vi "getConfiguration.vi"(8 "error in (no error)":errorcluster, 11 "Xcite in":refnum<class "Xcite.lvclass">) -> (0 "error out":errorcluster, 2 "configuration":cluster{"intensities":u32[], "on_states":u8[]}, 3 "Xcite out":refnum<class "Xcite.lvclass">)   [LabVIEW 2019, in "Xcite.lvclass"]
doc: "Returns the on/off state and intensity of each channel."
uses:
  Xcite.lvclass
  Xcite.lvclass/Xcite.ctl
  etc.xcite/XCite.lvlib
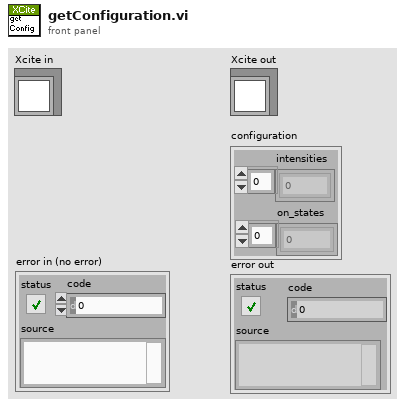
[diagram p1: front panel]
types:
  T1 = cluster{"LightSourceName":string, "hDevice":u64, "hCamera":u64, "iNumChannels":i32, "iNumWheels":i32, "dwSystemState":u32, "dwSerialNumber":u32, "dwSystemCaps":u32, "iLastChannelOnWheel":i16[], "XCiteChannels":cluster{"szLedName":string, "iWaveLength":i32, "IBelongToWheelNumber":i32, "iIntensity":i32, "iIntensityMin":i32, "iIntensityMax":i32, "iIntensityStep":i32, "iExtTriggerNum":i32, "iLedTemp":i32, "dwLEDState":u32}[]}
  T2 = cluster{"szLedName":string, "iWaveLength":i32, "IBelongToWheelNumber":i32, "iIntensity":i32, "iIntensityMin":i32, "iIntensityMax":i32, "iIntensityStep":i32, "iExtTriggerNum":i32, "iLedTemp":i32, "dwLEDState":u32}[]
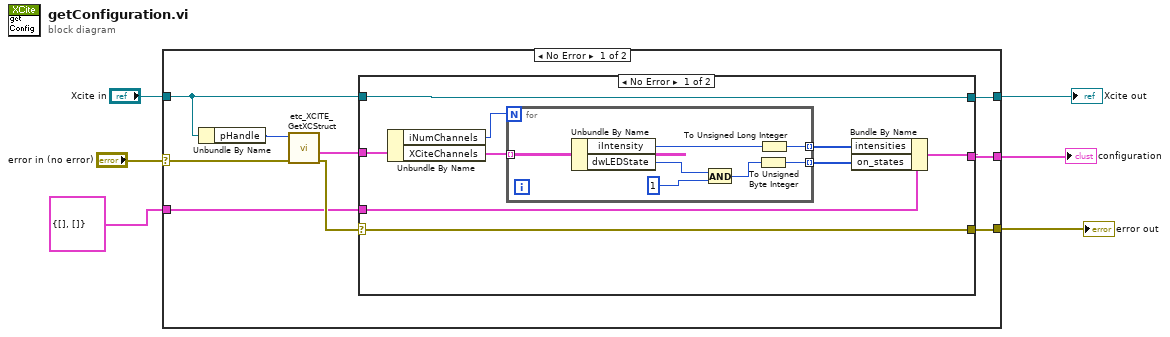
[diagram p0: block diagram]
diagram:
  n1 = case shown="No Error" "error in (no error)" {
    selector: "error in (no error)" -> [w14 w37]
    tunnel: [w11 w37] -> w5
    tunnel: "Xcite in" -> [w12 w36]
    tunnel: [w9 w36] -> w3
    tunnel: [w7 w35] -> w2
    tunnel: cluster{"intensities":u32[], "on_states":u8[]} {"intensities"=[], "on_states"=[]} ("XCITE_Configuration") -> [w8 w35]
    frame No Error {
      n2 = Unbundle By Name(w12) -> ("pHandle"=w15:u64)
      n3 = call "etc_XCITE_GetXCStruct.vi"("error in (no error)"=w14, "h"=w15) -> ("error out"=w13:errorcluster, "XCiteStructure"=w10:T1)  [unwired: 6 in, 2 out]
      n4 = case shown="No Error" w13 {
        selector: w13 -> [w23 w34]
        tunnel: w12 -> [w21 w33]
        tunnel: [w23 w34] -> w11
        tunnel: w10 -> [w22 _]
        tunnel: [w21 w33] -> w9
        tunnel: w8 -> [w20 w32]
        tunnel: [w17 w32] -> w7
        frame No Error {
          n5 = Unbundle By Name(w22) -> ("iNumChannels"=w16:i32, "XCiteChannels"=w24:T2)
          n6 = for {
            N: w16 -> [_]
            tunnel: w24 -> [w31] mode=indexing
            tunnel: [w25] -> w19 mode=indexing
            tunnel: [w26] -> w18 mode=indexing
            n7 = Unbundle By Name(w31) -> ("iIntensity"=w30:i32, "dwLEDState"=w29:u32)
            n8 = And(x=w29, y=u32 1) -> (x .and. y?=w27:u32)
            n9 = To Unsigned Byte Integer(number=w27) -> (unsigned 8bit integer=w26:u8)
            n10 = To Unsigned Long Integer(number=w30) -> (unsigned 32bit integer=w25:u32)
          }
          n11 = Bundle By Name(cluster=w20, "intensities"=w19, "on_states"=w18) -> (w17:cluster{"intensities":u32[], "on_states":u8[]})
        }
        frame Error {
        }
      }
    }
    frame Error {
    }
  }
  "Xcite out" <- w3
  "error out" <- w5
  "configuration" <- w2
